vi "RMYoung Anemometer.vi"   [LabVIEW 2014]
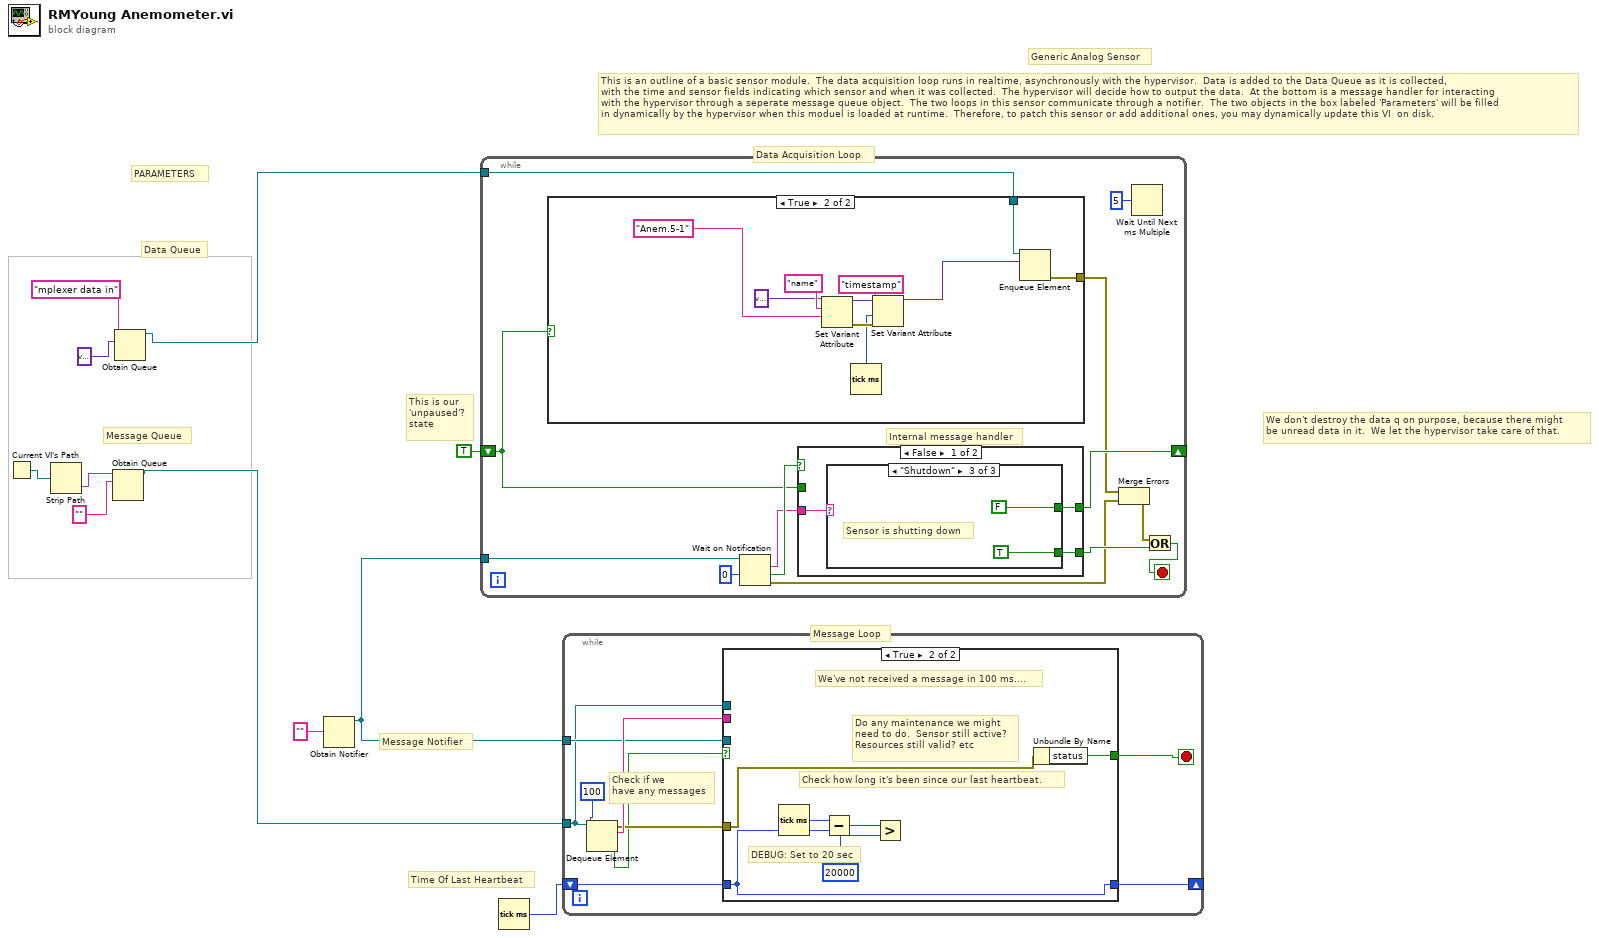
[diagram p0: block diagram]
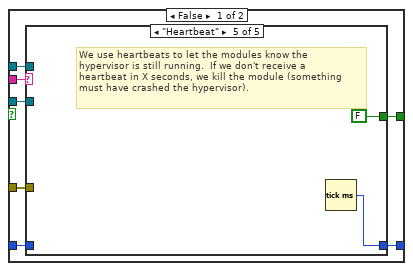
[diagram p2: hidden frame]
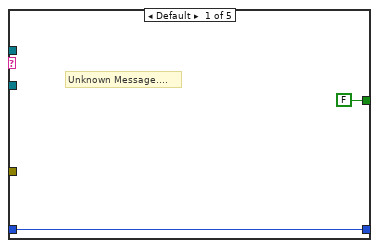
[diagram p3: hidden frame]
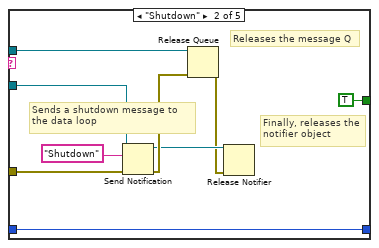
[diagram p4: hidden frame]
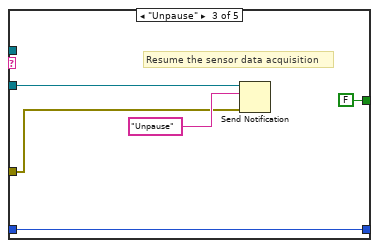
[diagram p5: hidden frame]
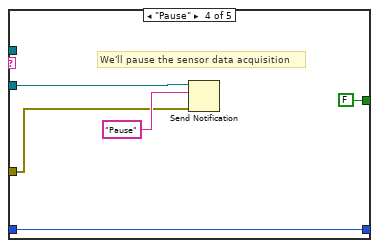
[diagram p6: hidden frame]
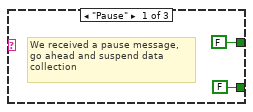
[diagram p8: hidden frame]
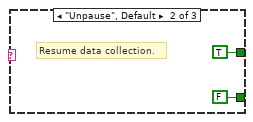
[diagram p9: hidden frame]
diagram:
  # "Time Of Last Heartbeat"
  # "This is an outline of a basic sensor module.  The data acquisition loop runs in realtime, asynchronously with the hypervisor.  Data is added to the Data Queue as it is collected,\nwith the time and sensor fields indicating which sensor and when it was collected.  The hypervisor will decide how to output the data.  At the bottom is a message handler for interacting\nwith the hypervisor through a seperate message queue object.  The two loops in this sensor communicate through a notifier.  The two objects in the box labeled 'Parameters' will be filled\nin dynamically by the hypervisor when this moduel is loaded at runtime.  Therefore, to patch this sensor or add additional ones, you may dynamically update this VI  on disk."
  # "This is our\n'unpaused'?\nstate"
  # "We don't destroy the data q on purpose, because there might\nbe unread data in it.  We let the hypervisor take care of that."
  # "Data Acquisition Loop"
  # "Message Loop"
  # "Message Notifier"
  # "Message Queue"
  # "Data Queue"
  # "PARAMETERS"
  # "Generic Analog Sensor"
  n1 = Current VI's Path() -> (path=w7:path)
  n2 = Strip Path(path=w7) -> (name=w6:string)  [unwired: 1 out]
  n3 = Obtain Queue(name (unnamed)=w6, element data type="") -> (queue out=w4:refnum<queue>)  [unwired: 3 in, 2 out]
  n4 = Obtain Queue(name (unnamed)="mplexer data in", element data type=variant) -> (queue out=w3:refnum<queue>)  [unwired: 3 in, 2 out]
  n5 = Obtain Notifier(notification data type="") -> (notifier out=w8:refnum<notifier>)  [unwired: 3 in, 2 out]
  n6 = while {
    tunnel: w3 -> [w16]
    tunnel: w8 -> [w24]
    shift-right: [w20] -> _
    shift-left: TRUE -> [w19]
    stop <- w15 stop-if-true
    # "Internal message handler"
    n7 = case shown="True" w19 {
      tunnel: w16 -> [_ w34]
      tunnel: [_ w33] -> w14
      frame False {
      }
      frame True {
        n8 = Set Variant Attribute(Variant=variant, name="name", value="Anem.5-1" ("Sensor Name")) -> (Variant out=w29:variant, error out=w30:errorcluster)  [unwired: 1 in, 1 out]
        n9 = Tick Count (ms)() -> (millisecond timer value=w27:u32)
        n10 = Set Variant Attribute(Variant=w29, name="timestamp", value=w27, error in=w30) -> (Variant out=w26:variant)  [unwired: 2 out]
        n11 = Enqueue Element(queue=w34, element=w26) -> (error out=w33:errorcluster)  [unwired: 2 in, 2 out]
      }
    }
    n12 = Wait on Notification(notifier=w24, timeout in ms (-1)=0) -> (notification=w21:string, timed out?=w22:bool, error out=w13:errorcluster)  [unwired: 2 in, 1 out]
    n13 = case shown="False" w22 {
      tunnel: w21 -> [w37 _]
      tunnel: [w36 _] -> w18
      tunnel: [w35 w44] -> w20
      tunnel: w19 -> [_ w44]
      frame False {
        n14 = case shown="\"Shutdown\"" w37 {
          tunnel: [FALSE FALSE TRUE] -> w36
          tunnel: [FALSE TRUE FALSE] -> w35
          frame "Pause" {
            # "We received a pause message,\ngo ahead and suspend data collection"
          }
          frame "Unpause", Default {
            # "Resume data collection."
          }
          frame "Shutdown" {
            # "Sensor is shutting down"
          }
        }
      }
      frame True {
      }
    }
    n15 = Merge Errors(w14, w13) -> (w12:errorcluster)
    n16 = Wait Until Next ms Multiple(millisecond multiple=u32 5) -> ()  [unwired: 1 out]
    n17 = Or(x=w12, y=w18) -> (x .or. y?=w15:bool)
  }
  n18 = Tick Count (ms)() -> (millisecond timer value=w9:u32)
  n19 = while {
    tunnel: w4 -> [w50]
    tunnel: w8 -> [w51]
    shift-right: [w45] -> _
    shift-left: w9 -> [w46]
    stop <- w52 stop-if-true
    # "Check if we \nhave any messages"
    n20 = Dequeue Element(queue=w50, timeout in ms (-1)=100) -> (element=w53:string, timed out?=w47:bool, error out=w49:errorcluster)  [unwired: 1 in, 1 out]
    n21 = case shown="True" w47 {
      tunnel: w53 -> [w60 _]
      tunnel: [w59 w84] -> w52
      tunnel: w51 -> [w58 _]
      tunnel: w50 -> [w57 _]
      tunnel: w49 -> [w56 w85]
      tunnel: w46 -> [w55 w86]
      tunnel: [w54 w86] -> w45
      frame False {
        n22 = case shown="\"Heartbeat\"" w60 {
          tunnel: [FALSE TRUE FALSE FALSE FALSE] -> w59
          tunnel: w58 -> [_ w69 w74 w78 _]
          tunnel: w57 -> [_ w70 _ _ _]
          tunnel: w56 -> [_ w68 w75 w79 _]
          tunnel: w55 -> [w61 w63 w72 w77 _]
          tunnel: [w61 w63 w72 w77 w83] -> w54
          frame Default {
            # "Unknown Message...."
          }
          frame "Shutdown" {
            # "Finally, releases the\nnotifier object"
            # "Releases the message Q"
            # "Sends a shutdown message to \nthe data loop"
            n23 = Send Notification(notification="Shutdown", notifier=w69, error in (no error)=w68) -> (notifier out=w65:refnum<notifier>, error out=w67:errorcluster)
            n24 = Release Queue(queue=w70, error in (no error)=w67) -> (error out=w64:errorcluster)  [unwired: 1 in, 2 out]
            n25 = Release Notifier(notifier=w65, error in (no error)=w64) -> ()  [unwired: 1 in, 3 out]
          }
          frame "Unpause" {
            # "Resume the sensor data acquisition"
            n26 = Send Notification(notification="Unpause", notifier=w74, error in (no error)=w75) -> ()  [unwired: 2 out]
          }
          frame "Pause" {
            # "We'll pause the sensor data acquisition"
            n27 = Send Notification(notification="Pause", notifier=w78, error in (no error)=w79) -> ()  [unwired: 2 out]
          }
          frame "Heartbeat" {
            # "We use heartbeats to let the modules know the \nhypervisor is still running.  If we don't receive a\nheartbeat in X seconds, we kill the module (something\nmust have crashed the hypervisor)."
            n28 = Tick Count (ms)() -> (millisecond timer value=w83:u32)
          }
        }
      }
      frame True {
        # "DEBUG: Set to 20 sec"
        # "Check how long it's been since our last heartbeat."
        # "Do any maintenance we might\nneed to do.  Sensor still active?\nResources still valid? etc"
        # "We've not received a message in 100 ms...."
        n29 = Tick Count (ms)() -> (millisecond timer value=w89:u32)
        n30 = Subtract(x=w89, y=w86) -> (x-y=w88:u32)
        n31 = Greater?(x=w88, y=u32 20000) -> ()  [unwired: 1 out]
        n32 = Unbundle By Name(w85) -> ("status"=w84:bool)
      }
    }
  }
